vi "FdxCmdFreeMemoryCvi.vi"(8 "error in":errorcluster, 11 "Mem":u32) -> (0 "error out":errorcluster)   [LabVIEW 2020, in "AIM664LV.lvlib"]
uses:
  AIM664LV.lvlib
  AFDX_LibraryAdmin/FdxGlobalDllPath.vi
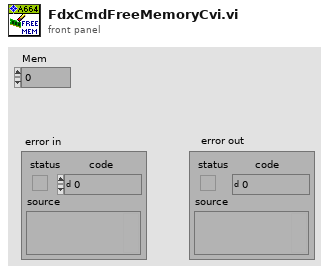
[diagram p1: front panel]
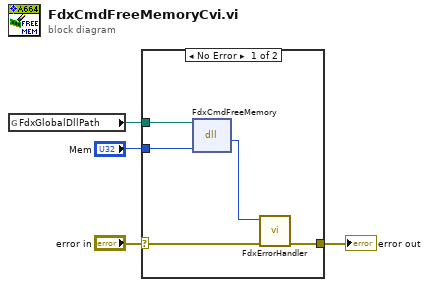
[diagram p0: block diagram]
diagram:
  n1 = global read "FdxGlobalDllPath.vi" "FdxGlobalDllPath"() -> (w2:path)
  n2 = case shown="No Error" "error in" {
    selector: "error in" -> [w8 w10]
    tunnel: [w9 w10] -> w4
    tunnel: w2 -> [w6 _]
    tunnel: "Mem" -> [w5 _]
    frame No Error {
      n3 = dll-call lib="aim_fdx.19.dll" fn="FdxCmdFreeMemory"(path in=w6, "Mem"=w5) -> ("status"=w7:i32)  [unwired: 3 in, 2 out]
      n4 = call "FdxErrorHandler.vi"("error in"=w8, "AIM Error"=w7) -> ("error out"=w9:errorcluster)  [unwired: 9 in]
    }
    frame Error {
    }
  }
  "error out" <- w4
